vi "fft2.vi"() -> ()   [LabVIEW 2014]
uses:
  <vilib>/Analysis/2dsp.llb/Real FFT.vi
  <vilib>/Waveform/WDTOps.llb/WDT Get XY Value DBL.vi
  <vilib>/Analysis/NI_AALPro.lvlib
  <vilib>/Analysis/NI_AALBase.lvlib
panel:
  in  "Stop":bool
  out "No":bool
  in  "Y position":dbl format="%0.0f"
  out "Y value":dbl format="%0.2f"
  out "actual Y position":dbl format="%0.2f"
  out "Yes":bool
  out "Test":cluster{dbl[], dbl[]}[](graph)
  in  "Low":dbl
  in  "High":dbl
  in  "Left":dbl
  in  "Right":dbl
  out "max value":dbl
  in  "fs (Hz)":dbl=1000.0 format="%#_13g"
  in  "Amplitude":dbl=1.0 format="%0.2f"
  out "Sine":dbl[](graph)
  out "FFT":dbl[](graph)
  in  "f0 (Hz)":dbl=0.0078125
  in  "FFT size":i32=-1
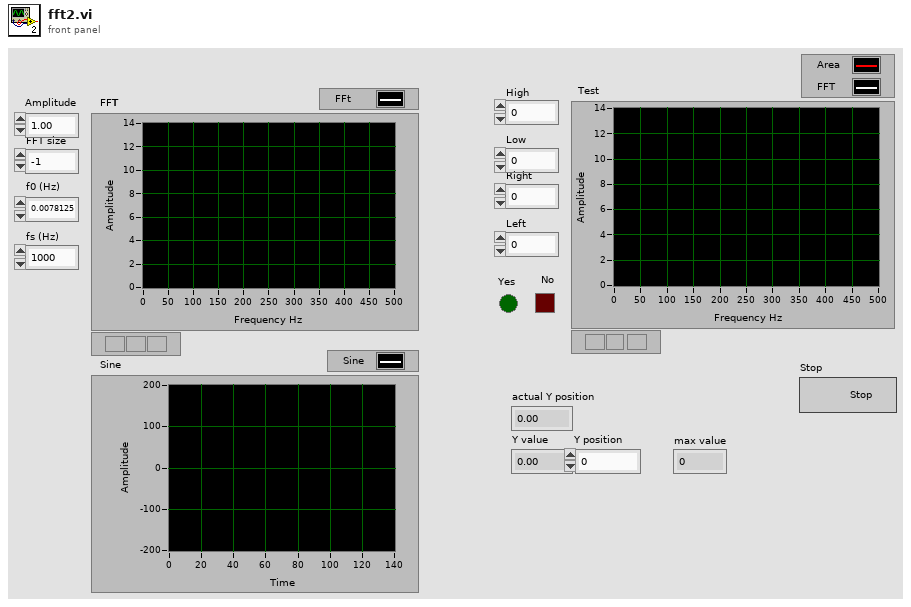
[diagram p1: front panel]
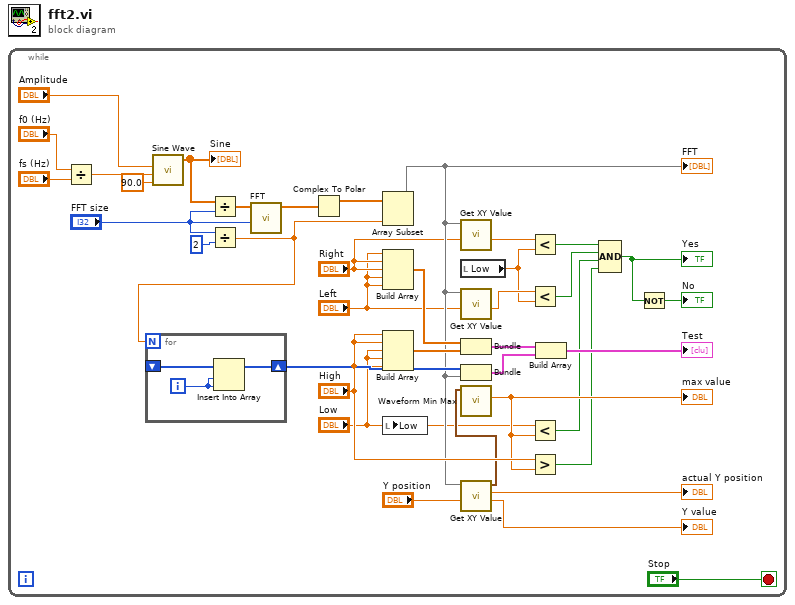
[diagram p0: block diagram]
diagram:
  n1 = while {
    stop <- "Stop" stop-if-true
    n2 = Divide(x="f0 (Hz)", y="fs (Hz)") -> (x/y=w34:dbl)
    n3 = call <vilib>:"Sine Wave.vi"("amplitude"="Amplitude", "frequency"=w34, "phase in"=90.0) -> ("sine wave"=w19:dbl[])  [unwired: 2 in, 2 out]
    "Sine" <- w19
    n4 = Divide(x=w19, y="FFT size") -> (x/y=w18:dbl[])
    n5 = Divide(x="FFT size", y=2) -> (x/y=w4:dbl)
    n6 = for {
      N: w4 -> [_]
      shift-right: [w40] -> w26
      shift-left: _ -> [w39]
      i -> [w41]
      n7 = Insert Into Array(array=w39, index=w41, new element=w41) -> (w40:i32[])
    }
    n8 = call-poly <vilib>:"FFT.vi"("FFT size"="FFT size", "X"=w18) -> ("FFT {X}"=w33:cdb[])  [unwired: 8 in, 1 out]
    n9 = Complex To Polar(r * e^(i*theta)=w33) -> (r=w38:dbl[])  [unwired: 1 out]
    n10 = Array Subset(array=w38, length=w4) -> (w17:dbl[])  [unwired: 1 in]
    "FFT" <- w17
    n11 = Build Array("Left", "Right", "Right", "Left", "Left") -> (w30:dbl[])
    n12 = Build Array("High", "High", "Low", "Low", "High") -> (w31:dbl[])
    n13 = local write "Low"("Low") -> ()
    n14 = call-poly <vilib>:"Get XY Value.vi"("Y position"="Right", "waveform in"=w17) -> ("Y value"=w14:dbl)  [unwired: 5 in, 4 out]
    n15 = local read "Low"() -> (w11:dbl)
    n16 = call-poly <vilib>:"Get XY Value.vi"("Y position"="Left", "waveform in"=w17) -> ("Y value"=w12:dbl)  [unwired: 5 in, 4 out]
    n17 = Bundle(w30, w31) -> (w28:cluster{dbl[], dbl[]})  [unwired: 1 in]
    n18 = Bundle(w26, w17) -> (w29:cluster{i32[], dbl[]})  [unwired: 1 in]
    n19 = call-poly <vilib>:"Get XY Value.vi"("Y position"="Y position", "waveform in"=w17) -> ("Y value"=→"Y value":dbl, "actual Y position"=→"actual Y position":dbl, "waveform out"=w23:waveform(dbl))  [unwired: 5 in, 2 out]
    n20 = call <vilib>:"Waveform Min Max.vi"("waveform in"=w23) -> ("Y max"=w24:dbl)  [unwired: 5 in, 5 out]
    "max value" <- w24
    n21 = Less?(x=w14, y=w11) -> (x < y?=w10:bool)
    n22 = Less?(x=w12, y=w11) -> (x < y?=w9:bool)
    n23 = Less?(x="Low", y=w24) -> (x < y?=w8:bool)
    n24 = Greater?(x="High", y=w24) -> (0:w7:bool)
    n25 = Build Array(w28, w29) -> (→"Test":cluster{dbl[], dbl[]}[])
    n26 = Compound Arithmetic op=AND(w10, w9, w8, w7) -> (w5:bool)
    "Yes" <- w5
    n27 = Not(x=w5) -> (.not. x?=→"No":bool)
  }
